vi "WRP Load Lens Table.vi"(8 "error in (no error)":errorcluster, 10 "filepath":string, 11 "lensmode":string) -> (0 "error out":errorcluster, 3 "function return":i32)   [LabVIEW 2018, in "SesWrapper.lvlib"]
doc: "int STDCALL WRP_SetPropertyDouble(const String property, int index, const double *value);"
uses:
  SesWrapper.lvlib
  build/Debug/SESWrapper.dll
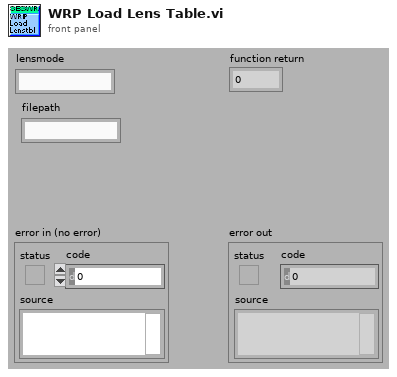
[diagram p1: front panel]
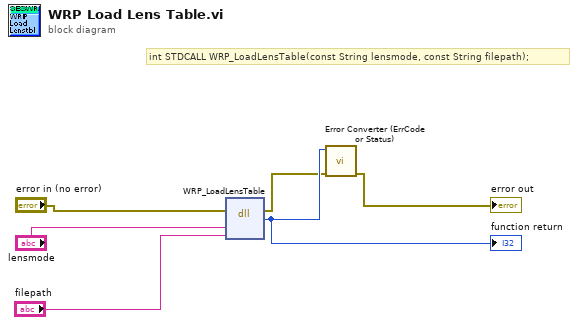
[diagram p0: block diagram]
diagram:
  # "int STDCALL WRP_LoadLensTable(const String lensmode, const String filepath);"
  n1 = dll-call lib="C:/Development/svn/seswrapper-lib/build/Debug/SESWrapper.*" fn="WRP_LoadLensTable" ("SESWrapper.dll:WRP_SetPropertyDouble")(error in="error in (no error)", "lensmode"="lensmode", "filepath"="filepath") -> (error out=w3:errorcluster, "return type"=w6:i32)  [unwired: 4 in, 1 out]
  "function return" <- w6
  n2 = call "Error Converter (ErrCode or Status).vi"("error in (no error)"=w3, "error code"=w6) -> ("error out"=→"error out":errorcluster)  [unwired: 9 in]
